vi "Is a Valid Number (DBL).vi"(2 "Number":dbl) -> (7 "Valid Number?":bool)   [LabVIEW 2021]
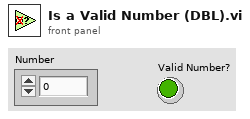
[diagram p1: front panel]
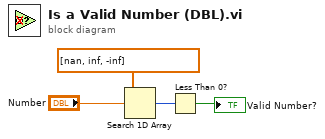
[diagram p0: block diagram]
diagram:
  n1 = Search 1D Array(1D array=dbl[] [nan, inf, -inf], element="Number") -> (index of element=w3:i32)  [unwired: 1 in]
  n2 = Less Than 0?(x=w3) -> (x < 0?=→"Valid Number?":bool)
